vi "ReadSamples.vi"(8 "error in (no error)":errorcluster, 9 "Max num samples to keep":u32, 10 "Num samples to read":u32, 11 "FpgaRef5761 In":refnum<class "FpgaRef5761.lvclass">) -> (0 "error out":errorcluster, 2 "Data":dbl[][](array[numeric]), 3 "FpgaRef5761 Out":refnum<class "FpgaRef5761.lvclass">)   [LabVIEW 2018, in "FpgaRef5761.lvclass"]
uses:
  FpgaRef5761.lvclass
  FpgaRef5761.lvclass/FpgaRef5761.ctl
  <vilib>/Utility/error.llb/Error Cluster From Error Code.vi
  <vilib>/rvi/errors/niLvFpgaAdjustHostInterfaceError.vi
  <vilib>/rvi/interface/nirviMethod/nirviMethod.xnode
  5761 FPGA ref.ctl
  <vilib>/FPGAPlugInAG/Dynamic/niLvFpga_AcquireReadRegionFifo_Dynamic.vi
  <vilib>/rvi/errors/niLvFpgaMergeErrorWithErrorCode.vi
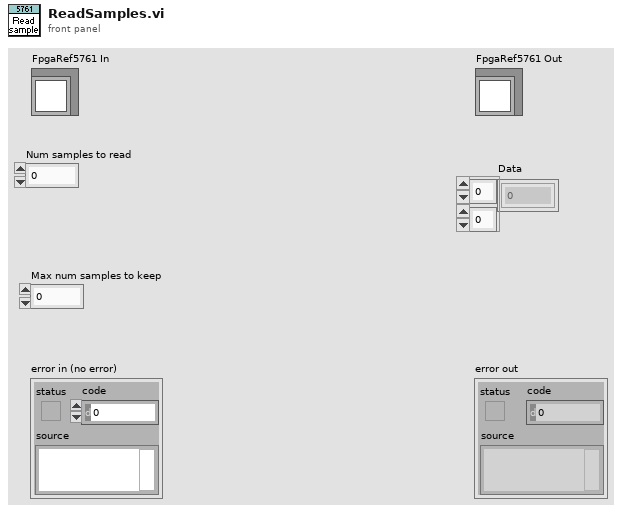
[diagram p1: front panel]
types:
  T1 = typedef "5761 FPGA ref.ctl" = refnum<k20>
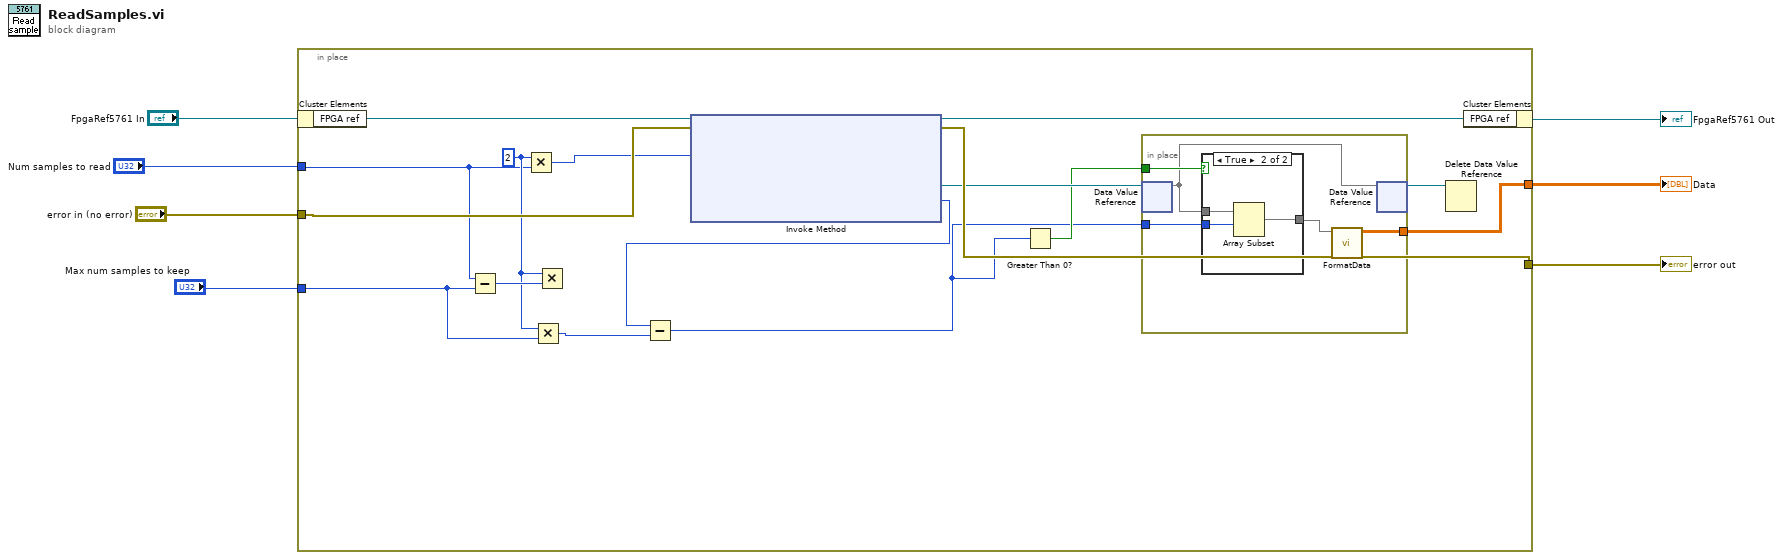
[diagram p0: block diagram]
diagram:
  n1 = in-place {
    in-place-border: [w14] -> w5
    in-place-border: [w19] -> w2
    in-place-border: "Num samples to read" -> [w11]
    in-place-border: "error in (no error)" -> [w22]
    in-place-border: "Max num samples to keep" -> [w12]
    w13 = u32 2 ("x")
    n2 = in-place-cluster #1("FpgaRef5761 In") -> ("FPGA ref"=w21:T1)
    n3 = Subtract(x=w11, y=w12) -> (x-y=w23:u32)
    n4 = Multiply(x=w13, y=w11) -> (x*y=w18:u32)
    n5 = Multiply(x=w13, y=w12) -> (x*y=w10:u32)
    n6 = Multiply(x=w13, y=w23) -> ()  [unwired: 1 out]
    n7 = xnode "Invoke Method"("FPGA VI Reference In"=w21, "error in"=w22, "Number of Elements"=w18) -> ("FPGA VI Reference Out"=w20:T1, "error out"=w19:errorcluster, "Read Region Reference"=w17:refnum<data-value>, "Elements In Region"=w9:u32)  [unwired: 1 in, 1 out]
    n8 = Subtract(x=w9, y=w10) -> (x-y=w8:u32)
    n9 = Greater Than 0?(x=w8) -> (x > 0?=w15:bool)
    n10 = in-place {
      in-place-border: w15 -> [w27]
      in-place-border: w8 -> [w26]
      in-place-border: [w25] -> w14
      n11 = in-place-dvr #2(w17) -> (w24:u64[])  [unwired: 1 out]
      n12 = case shown="True" w27 {
        tunnel: w24 -> [w29 w32]
        tunnel: w26 -> [_ w31]
        tunnel: [w29 w30] -> w28
        frame False {
        }
        frame True {
          n13 = Array Subset(array=w32, index=w31) -> (w30:u64[])  [unwired: 1 in]
        }
      }
      n14 = call "FormatData.vi"("Raw data"=w28) -> ("Scaled"=w25:dbl[][])  [unwired: 10 in]
      n15 = in-place-dvr #2(w24) -> (w16:refnum<data-value>)  [unwired: 1 out]
    }
    n16 = Delete Data Value Reference(data value reference=w16) -> ()  [unwired: 1 in, 2 out]
    n17 = in-place-cluster #1("FPGA ref"=w20) -> (→"FpgaRef5761 Out":refnum<class "FpgaRef5761.lvclass">)
  }
  "error out" <- w2
  "Data" <- w5
